vi "Revision Query.vi"(8 "error in (no error)":errorcluster, 11 "VISA resource name":refnum<visa-resource-name>) -> (0 "error out":errorcluster, 1 "Instrument Firmware Revision":string, 2 "Instrument Driver Revision":string, 3 "VISA resource name out":refnum<visa-resource-name>)   [LabVIEW 2009, in "Tektronix DPO MSO 2000 4000 Series.lvlib"]
doc: "Queries the current revision of the instrument firmware and instrument drivers.\n\nRefer to the Readme for information about instrument drivers, including information about modification history."
uses:
  <instrlib>/Tektronix DPO MSO 2000 4000 Series/Tektronix DPO MSO 2000 4000 Series.lvlib
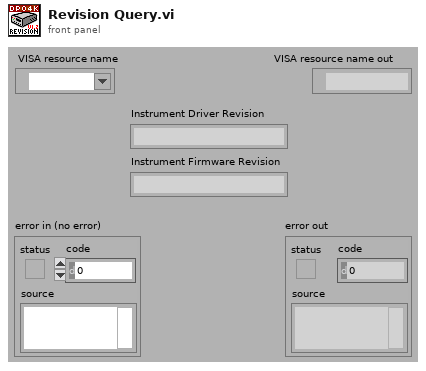
[diagram p1: front panel]
types:
  T1 = enum32{"invalid app kind", "Development System", "Run Time System", "Student Edition", "Embedded LabVIEW", "Evaluation", "Custom"}
  T2 = cluster{"Major":u16, "Minor":u16, "Fix":u16, "Build":u16}
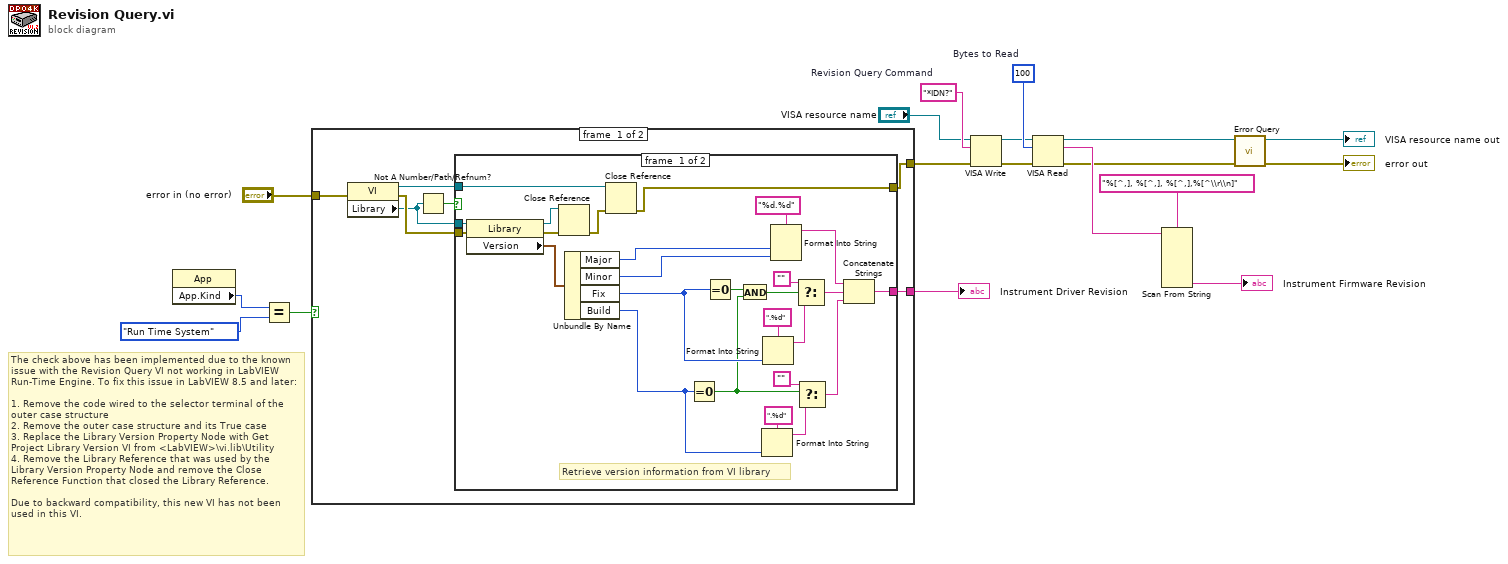
[diagram p0: block diagram]
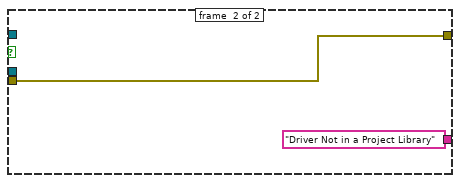
[diagram p2: hidden frame]
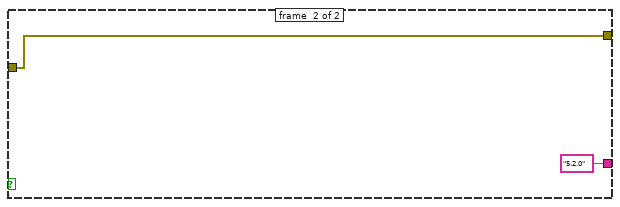
[diagram p3: hidden frame]
diagram:
  w15 = "*IDN?"  # Revision Query Command
  w18 = u32 100  # Bytes to Read
  # "The check above has been implemented due to the known issue with the Revision Query VI not working in LabVIEW Run-Time Engine. To fix this issue in LabVIEW 8.5 and later:\n\n1. Remove the code wired to the selector terminal of the outer case structure\n2. Remove the outer case structure and its True case\n3. Replace the Library Version Property Node with Get Project Library Version VI from <LabVIEW>\\vi.lib\\Utility\n4. Remove the Library Reference that was used by the Library Version Property Node and remove the Close Reference Function that closed the Library Reference.\n\nDue to backward compatibility, this new VI has not been used in this VI."
  n1 = property class="App"() -> ("App.Kind"=w8:T1)  [unwired: 2 in, 2 out]
  n2 = Equal?(x=w8, y=T1."Run Time System" ("Application:Kind")) -> (x = y?=w9:bool)
  n3 = case shown="False" w9 {
    tunnel: [w21 "5.2.0"] -> w1
    tunnel: [w20 w54] -> w10
    tunnel: "error in (no error)" -> [w19 w54]
    frame #0 {
      n4 = property class="VI"(error in=w19) -> (reference out=w25:refnum<vi>, error out=w24:errorcluster, "Library"=w23:refnum<vi>)  [unwired: 1 in]
      n5 = Not A Number/Path/Refnum?(number/path/refnum=w23) -> (NaN/Path/Refnum?=w22:bool)
      n6 = case shown="False" w22 {
        tunnel: w25 -> [w48 _]
        tunnel: w24 -> [w33 w53]
        tunnel: [w28 w53] -> w20
        tunnel: [w27 "Driver Not in a Project Library"] -> w21
        tunnel: w23 -> [w26 _]
        frame #0 {
          # "Retrieve version information from VI library"
          n7 = property class="Library"(reference=w26, error in=w33) -> (reference out=w50:refnum<vi>, error out=w51:errorcluster, "Version"=w47:T2)
          n8 = Close Reference(reference=w50, error in (no error)=w51) -> (error out=w49:errorcluster)
          n9 = Unbundle By Name(w47) -> ("Major"=w36:u16, "Minor"=w35:u16, "Fix"=w32:u16, "Build"=w34:u16)
          n10 = Close Reference(reference=w48, error in (no error)=w49) -> (error out=w28:errorcluster)
          n11 = Equal To 0?(x=w34) -> (x = 0?=w30:bool)
          n12 = Equal To 0?(x=w32) -> (x = 0?=w31:bool)
          n13 = And(x=w31, y=w30) -> (x .and. y?=w29:bool)
          n14 = Format Into String(format string=".%d", w34) -> (resulting string=w40:string)  [unwired: 2 in, 1 out]
          n15 = Format Into String(format string=".%d", w32) -> (resulting string=w44:string)  [unwired: 2 in, 1 out]
          n16 = Format Into String(format string="%d.%d", w36, w35) -> (resulting string=w42:string)  [unwired: 2 in, 1 out]
          n17 = Select(t="", s=w29, f=w44) -> (s? t:f=w41:string)
          n18 = Select(t="", s=w30, f=w40) -> (s? t:f=w37:string)
          n19 = Concatenate Strings(w42, w41, w37) -> (w27:string)
        }
        frame #1 {
        }
      }
    }
    frame #1 {
    }
  }
  "Instrument Driver Revision" <- w1
  n20 = VISA Write(VISA resource name="VISA resource name", write buffer=w15, error in (no error)=w10) -> (VISA resource name out=w17:refnum<visa-resource-name>, error out=w16:errorcluster)  [unwired: 1 out]
  n21 = VISA Read(VISA resource name=w17, byte count=w18, error in (no error)=w16) -> (VISA resource name out=w11:refnum<visa-resource-name>, read buffer=w14:string, error out=w12:errorcluster)  [unwired: 1 out]
  n22 = Scan From String(format string="%[^,], %[^,], %[^,],%[^\\r\\n]", input string=w14) -> (output 4=→"Instrument Firmware Revision":string)  [unwired: 9 in, 3 out]
  n23 = call <instrlib>:"Error Query.vi"("error in (no error)"=w12, "VISA resource name"=w11) -> ("error out"=→"error out":errorcluster, "VISA resource name out"=→"VISA resource name out":refnum<visa-resource-name>)  [unwired: 6 in, 2 out]
